vi "SGL_to_U32.vi"(1 "SGL":sgl) -> (4 "U32":u32)   [LabVIEW 2016]
uses:
  <vilib>/rvi/IPIntegrationNode/IPINode_Xnode/niFpgaIPINode.xnode
  typecast_SGL_to_U32SimFiles/xsim.dir/typecast_SGL_to_U32/xsimkE139BA94F1564A7E9F64A34773DA2B61.dll
  <vilib>/rvi/IPIntegrationNode/IPINode_Typedef/niFpgaIPINodeSupportedFamilies.ctl
  <vilib>/rvi/IPIntegrationNode/IPINode_Utilities/niFpgaIPINodeSimCore.vi
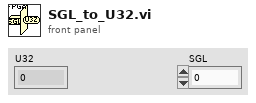
[diagram p1: front panel]
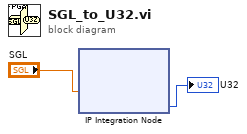
[diagram p0: block diagram]
diagram:
  n1 = xnode ("IP Integration Node")("sgl"="SGL") -> ("u32"=→"U32":u32)
